vi "Convert Signal List to Array.vi"(11 "Signal List":string) -> (3 "Signal List":string[](array[string]))   [LabVIEW 2025, in "Signal.lvclass"]
doc: "Script Input Signal IP."
uses:
  Signal.lvclass
  <vilib>/Utility/error.llb/Trim Whitespace One-Sided.vi
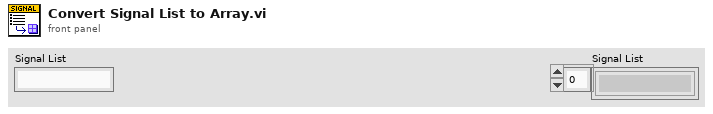
[diagram p1: front panel]
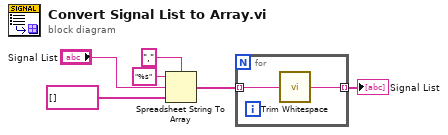
[diagram p0: block diagram]
diagram:
  n1 = Spreadsheet String To Array(delimiter (Tab)=",", format string="%s", spreadsheet string="Signal List", array type (2D Dbl)=string[] []) -> (array=w3:string[])
  n2 = for {
    tunnel: w3 -> [w8] mode=indexing
    tunnel: [w7] -> w1 mode=indexing
    n3 = call <vilib>:"Trim Whitespace.vi"("string"=w8) -> ("trimmed string"=w7:string)  [unwired: 1 in]
  }
  "Signal List" <- w1
